vi "Configure Multi Eval Meas Modulation EVM Symbol.vi"(6 "Position (Low)":i32(ring) items=["Low", "High"], 7 "Symbol (0)":i32, 8 "error in (no error)":errorcluster, 9 "Enabled (Off)":bool, 10 "Instance (1)":T1=1, 11 "VISA resource name":refnum<visa-resource-name>) -> (0 "error out":errorcluster, 3 "VISA resource name out":refnum<visa-resource-name>)   [LabVIEW 2020, in "Rohde&Schwarz CMWXP NR FR1 Measurement.lvlib"]
doc: "Enables or disables the measurement of EVM vs modulation symbol results and configures the scope of the measurement.\n\nAttribute:\nRSCMWXPNRFR1M_ATTR_MULTI_EVAL_MEAS_MODULATION_EVM_SYMBOL_RESULT\n\nRemote-control command:\nCONFigure:NRSub:MEAS<i>:MEValuation:RESult:EVMagnitude:EVMSymbol"
uses:
  <instrlib>/Rohde&Schwarz CMWXP NR FR1 Measurement/Rohde&Schwarz CMWXP NR FR1 Measurement.lvlib
  <instrlib>/Rohde&Schwarz CMWXP NR FR1 Measurement/Private/_Instance.ctl
  <instrlib>/Rohde&Schwarz CMWXP NR FR1 Measurement/Private/rsidr_core.llb/rsidr_core.lvlib
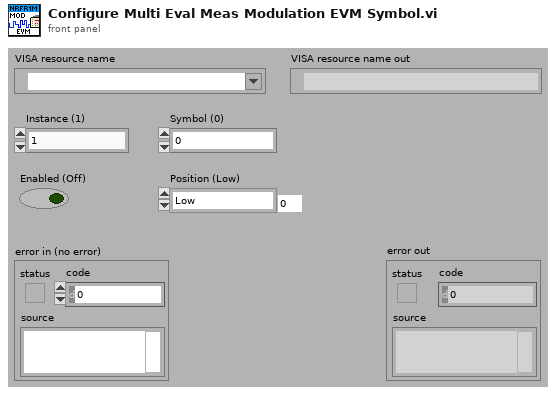
[diagram p1: front panel]
types:
  T1 = typedef "Rohde&Schwarz CMWXP NR FR1 Measurement.lvlib/_Instance.ctl" = i32
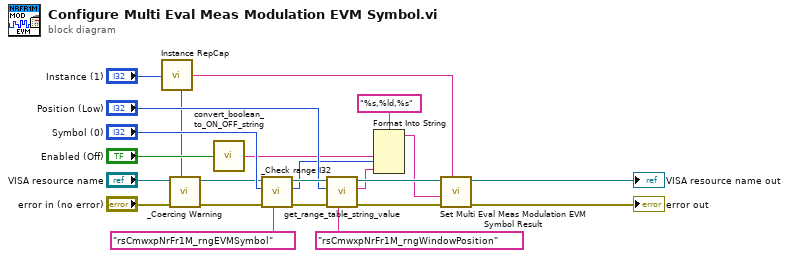
[diagram p0: block diagram]
diagram:
  n1 = call <instrlib>:"Instance RepCap.vi"("Instance In"="Instance (1)") -> ("In Range?"=w1:bool, "RepCap Identifier Out"=w22:string)  [unwired: 1 in]
  n2 = call <instrlib>:"_Coercing Warning.vi"("In Range?"=w1, "error in (no error)"="error in (no error)", "VISA resource name"="VISA resource name") -> ("error out"=w3:errorcluster, "VISA resource name out"=w2:refnum<visa-resource-name>)  [unwired: 7 in]
  n3 = call <instrlib>:"convert_boolean_to_ON_OFF_string.vi"("boolean value in"="Enabled (Off)") -> ("string value out"=w9:string)  [unwired: 4 in]
  n4 = call <instrlib>:"_Check range I32.vi"("Range Table Identifier"="rsCmwxpNrFr1M_rngEVMSymbol", "error in (no error)"=w3, "I32 Value In"="Symbol (0)", "VISA resource name"=w2) -> ("error out"=w18:errorcluster, "I32 Value Out"=w8:i32, "VISA resource name out"=w17:refnum<visa-resource-name>)  [unwired: 5 in]
  n5 = call <instrlib>:"get_range_table_string_value.vi"("Range Table ID in"="rsCmwxpNrFr1M_rngWindowPosition", "error in"=w18, "I32 input"="Position (Low)", "VISA resource name"=w17) -> ("error out"=w16:errorcluster, "String Value out"=w7:string, "VISA resource name out"=w15:refnum<visa-resource-name>)  [unwired: 5 in]
  n6 = Format Into String(format string="%s,%ld,%s", w9, w8, w7) -> (resulting string=w6:string)  [unwired: 2 in, 1 out]
  n7 = call "Set Multi Eval Meas Modulation EVM Symbol Result"("Repeated Capabilities"=w22, "error in (no error)"=w16, "Multi Eval Meas Modulation EVM Symbol Result ()"=w6, "instrument handle"=w15) -> ("error out"=→"error out":errorcluster, "instrument handle out"=→"VISA resource name out":refnum<visa-resource-name>)  [unwired: 6 in]
